vi "[nc] Write Color.vi"(10 "Color":T1, 11 "Piece in":refnum<class "Piece.lvclass">) -> (3 "Piece out":refnum<class "Piece.lvclass">)   [LabVIEW 2016]
uses:
  Piece.lvclass
  typedef/Color.ctl
  Chesslib.lvlib
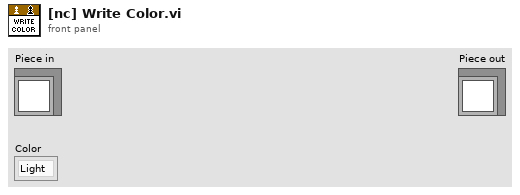
[diagram p1: front panel]
types:
  T1 = typedef "Chesslib.lvlib/Color.ctl" = enum16{"Light", "Dark"}
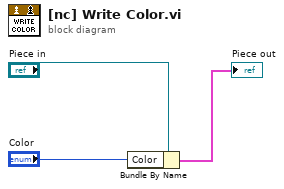
[diagram p0: block diagram]
diagram:
  n1 = Bundle By Name(cluster="Piece in", "Color"="Color") -> (→"Piece out":cluster{})
